vi "update_dust_event.vi"(7 "Small?":bool, 8 "error in (no error)":errorcluster, 11 "Cluster":T1 {"File Location" items=["Unknown"=-5, "IDL Processing"=-4, "Writing from Queue"=-3, "Labview Files"=-2, "Retry Labview files"=-1, "Local Cache "=0, "Storage"=1]}) -> (0 "error out":errorcluster)   [LabVIEW 2013]
uses:
  Public API/Post_Dust_Event.ctl
  Private/Controls/File_location.ctl
  <vilib>/addons/database/NI_Database_API.lvlib
panel:
  out "concatenated string":string
  # "Dust Event"
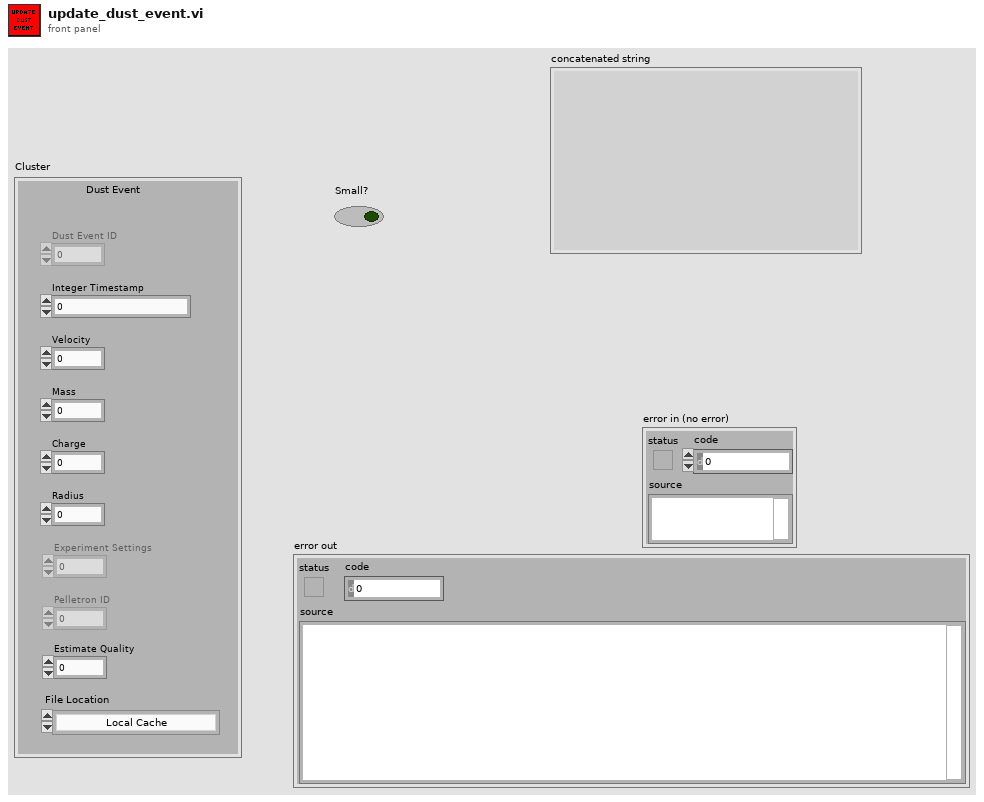
[diagram p1: front panel]
types:
  T1 = typedef "Post_Dust_Event.ctl" = cluster{"Dust Event ID":i64, "Integer Timestamp":i64, "Velocity":sgl, "Mass":sgl, "Charge":sgl, "Radius":sgl, "Experiment Settings":dbl, "Pelletron ID":i32, "Estimate Quality":sgl, "File Location":T2, "id_dust_info":dbl}
  T2 = typedef "File_location.ctl" = i8
  T3 = cluster{"Velocity":sgl, "Mass":sgl, "Charge":sgl, "Radius":sgl, "Estimate Quality":sgl}
  T4 = typedef "NI_Database_API.lvlib/Conn ObjectReference.ctl" = refnum<k1>
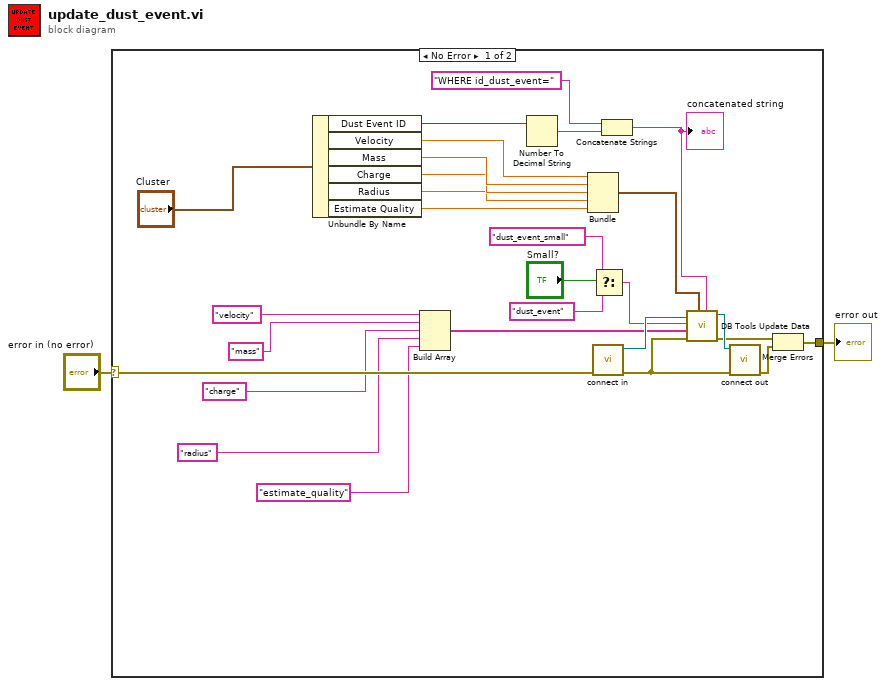
[diagram p0: block diagram]
diagram:
  n1 = case shown="No Error" "error in (no error)" {
    selector: "error in (no error)" -> [w29 w31]
    tunnel: [w26 w31] -> w1
    frame No Error {
      n2 = Unbundle By Name("Cluster") -> ("Dust Event ID"=w22:i64, "Velocity"=w7:sgl, "Mass"=w16:sgl, "Charge"=w15:sgl, "Radius"=w14:sgl, "Estimate Quality"=w13:sgl)
      n3 = Build Array("velocity" ("string"), "mass" ("string"), "charge" ("string"), "radius" ("string"), "estimate_quality" ("string")) -> (w17:string[])
      n4 = Number To Decimal String(number=w22) -> (decimal integer string=w19:string)  [unwired: 1 in]
      n5 = Bundle("Velocity"=w7, "Mass"=w16, "Charge"=w15, "Radius"=w14, "Estimate Quality"=w13) -> (w12:T3)  [unwired: 1 in]
      n6 = call "connect in.vi"("error in (no error)"=w29) -> ("error out"=w28:errorcluster, "Database Connection"=w30:T4)  [unwired: 6 in, 1 out]
      n7 = Select(t="dust_event_small" ("table"), s="Small?", f="dust_event" ("table")) -> (s? t:f=w4:string)
      n8 = Concatenate Strings("WHERE id_dust_event=" ("condition"), w19) -> (w21:string)
      "concatenated string" <- w21
      n9 = call <vilib>:"DB Tools Update Data.vi"("condition"=w21, "data"=w12, "error in (no error)"=w28, "columns"=w17, "table"=w4, "connection reference"=w30) -> ("error out"=w24:errorcluster, "connection reference out"=w25:T4)  [unwired: 4 in]
      n10 = call "connect out.vi"("error in (no error)"=w28, "connection reference"=w25) -> ("error out"=w27:errorcluster)  [unwired: 9 in]
      n11 = Merge Errors(w24, w27) -> (w26:errorcluster)
    }
    frame Error {
    }
  }
  "error out" <- w1
